vi "Get Publish IDs for Stepped Sine Frequence Response.vi"(8 "Error In":errorcluster, 11 "No of  Sweep Configurations":i32) -> (0 "Error Out":errorcluster, 3 "Publish IDs":tag[](array[tag]))   [LabVIEW 2020]
doc: "This Vi helps to generate Publish IDs for Stepped Sine Frequence Response"
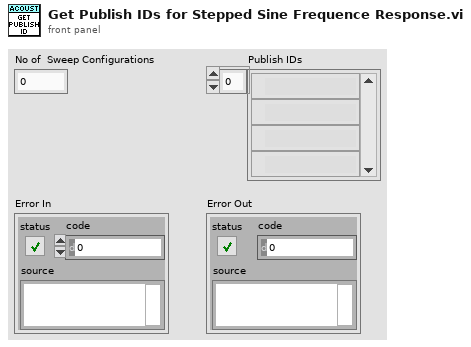
[diagram p1: front panel]
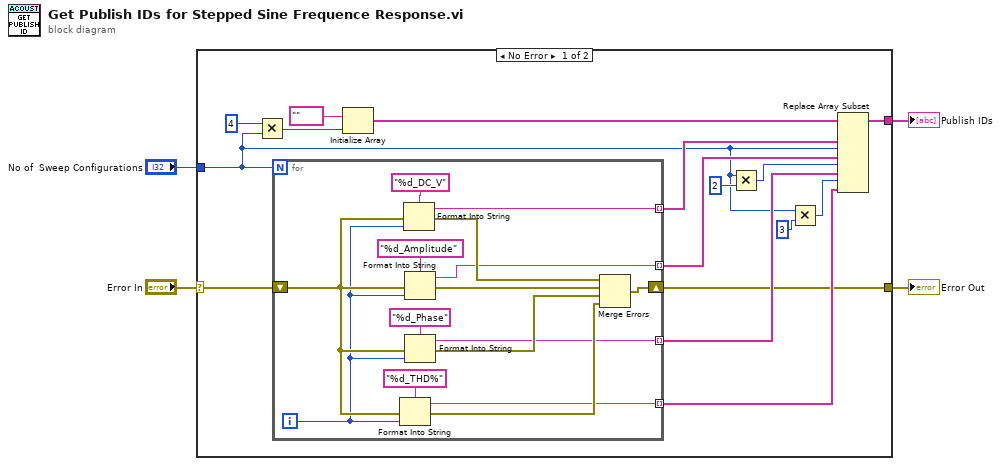
[diagram p0: block diagram]
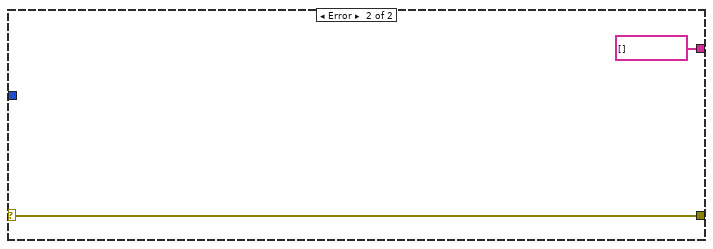
[diagram p2: hidden frame]
diagram:
  n1 = case shown="No Error" "Error In" {
    selector: "Error In" -> [w6 w36]
    tunnel: [w15 tag[] []] -> w4
    tunnel: "No of  Sweep Configurations" -> [w9 _]
    tunnel: [w5 w36] -> w1
    frame No Error {
      n2 = Multiply(x=4, y=w9) -> (x*y=w13:i32)
      n3 = for {
        N: w9 -> [_]
        shift-right: [w30] -> w5
        shift-left: w6 -> [w35]
        tunnel: [w24] -> w12 mode=indexing
        tunnel: [w23] -> w18 mode=indexing
        tunnel: [w22] -> w17 mode=indexing
        tunnel: [w21] -> w16 mode=indexing
        i -> [w25]
        n4 = Format Into String(format string="%d_THD%", error in=w35, w25) -> (resulting string=w21:string, error out=w31:errorcluster)  [unwired: 1 in]
        n5 = Format Into String(format string="%d_DC_V", error in=w35, w25) -> (resulting string=w24:string, error out=w34:errorcluster)  [unwired: 1 in]
        n6 = Format Into String(format string="%d_Amplitude", error in=w35, w25) -> (resulting string=w23:string, error out=w33:errorcluster)  [unwired: 1 in]
        n7 = Format Into String(format string="%d_Phase", error in=w35, w25) -> (resulting string=w22:string, error out=w32:errorcluster)  [unwired: 1 in]
        n8 = Merge Errors(w34, w33, w32, w31) -> (w30:errorcluster)
      }
      n9 = Initialize Array(tag "" ("Published Data Id"), w13) -> (w19:tag[])
      n10 = Multiply(x=w9, y=2) -> (x*y=w10:i32)
      n11 = Multiply(x=w9, y=3) -> (x*y=w7:i32)
      n12 = Replace Array Subset(array=w19, new element #1=w12, new element #2=w18, index #2=w9, new element #3=w17, index #3=w10, new element #4=w16, index #4=w7) -> (w15:tag[])  [unwired: 1 in]
    }
    frame Error {
    }
  }
  "Publish IDs" <- w4
  "Error Out" <- w1
